vi "Display and Log Custom Device Error.vi"(7 "Error Log Settings":T1, 8 "error out":errorcluster, 9 "Note (empty)":string, 10 "Your code's public name":string, 11 "Custom Device? (T)":bool=TRUE) -> ()   [LabVIEW 2026, in "VS Inline Async API (Express).lvlib" / "VS Inline Async API (Express).lvclass"]
uses:
  VS Inline Async API (Express).lvclass
  <vilib>/NI VeriStand/Custom Device Tools/Custom Device Utility Library/Custom Device Utility Library.lvlib
  VS Inline Async API (Express).lvlib
  <vilib>/Utility/SystemLogging/NI_SystemLogging.lvlib
  <vilib>/Utility/error.llb/Trim Whitespace (string).vi
  Types/Error Handling Settings.ctl
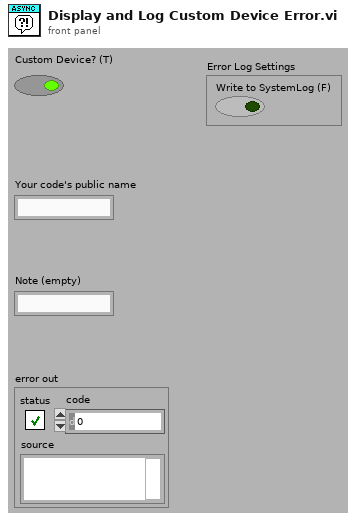
[diagram p1: front panel]
types:
  T1 = typedef "VS Inline Async API (Express).lvlib/VS Inline Async API (Express).lvclass/Error Handling Settings.ctl" = cluster{"Write to SystemLog (F)":bool}
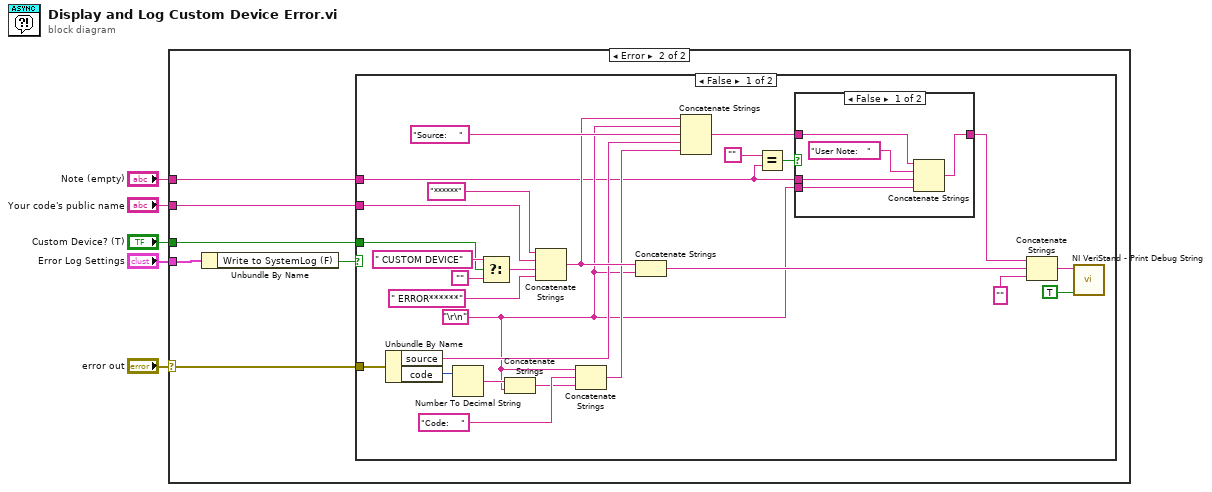
[diagram p0: block diagram]
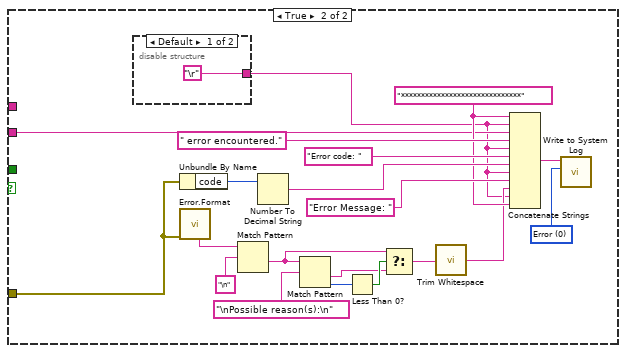
[diagram p4: hidden frame]
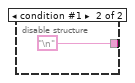
[diagram p5: hidden frame]
diagram:
  n1 = case shown="Error" "error out" {
    selector: "error out" -> [_ w11]
    tunnel: "Custom Device? (T)" -> [_ w10]
    tunnel: "Your code's public name" -> [_ w9]
    tunnel: "Note (empty)" -> [_ w8]
    tunnel: "Error Log Settings" -> [_ w7]
    frame No Error {
    }
    frame Error {
      n2 = Unbundle By Name(w7) -> ("Write to SystemLog (F)"=w6:bool)
      n3 = case shown="False" w6 {
        tunnel: w11 -> [w37 w46]
        tunnel: w10 -> [w25 _]
        tunnel: w9 -> [w16 w45]
        tunnel: w8 -> [w14 _]
        frame False {
          w15 = "\r\n"
          n4 = Unbundle By Name(w37) -> ("source"=w24:string, "code"=w18:i32)
          n5 = Number To Decimal String(number=w18) -> (decimal integer string=w34:string)  [unwired: 1 in]
          n6 = Select(t=" CUSTOM DEVICE" ("String"), s=w25, f="") -> (s? t:f=w26:string)
          n7 = Concatenate Strings(w34, w15) -> (w17:string)
          n8 = Concatenate Strings("******" ("String"), w16, w26, " ERROR******" ("String")) -> (w29:string)
          n9 = Concatenate Strings(w15, "Code:    " ("String"), w17) -> (w23:string)
          n10 = Concatenate Strings(w29, w15) -> (w20:string)
          n11 = Concatenate Strings(w29, w15, "Source:    " ("String"), w24, w23) -> (w22:string)
          n12 = Equal?(x="", y=w14) -> (x = y?=w27:bool)
          n13 = case shown="False" w27 {
            tunnel: w14 -> [w41 _]
            tunnel: w15 -> [w40 _]
            tunnel: w22 -> [w39 w43]
            tunnel: [w38 w43] -> w21
            frame False {
              n14 = Concatenate Strings(w39, "User Note:   " ("string"), w41, w40) -> (w38:string)
            }
            frame True {
            }
          }
          n15 = Concatenate Strings(w21, w20, "" ("Message")) -> (w13:string)
          n16 = call <vilib>:"NI VeriStand - Print Debug String.vi"("Add to log file? (F)"=TRUE ("Add to log file? (T)"), "Message"=w13) -> ()  [unwired: 9 in, 1 out]
        }
        frame True {
          w58 = "******************************" ("string")
          w63 = 0 items=["Error", "Warning", "Informational"] ("severity")
          n17 = disable-structure shown="Default" {
            disable-tunnel: ["\r" "\n"] -> w44
            frame condition #0 (active) {
            }
            frame condition #1 {
            }
          }
          n18 = Unbundle By Name(w46) -> ("code"=w47:i32)
          n19 = call "Error.Format.vi"("error in (no error)"=w46) -> ("message"=w48:string)  [unwired: 6 in, 4 out]
          n20 = Match Pattern(string=w48, regular expression="\n" ("string")) -> (after substring=w53:string)  [unwired: 1 in, 3 out]
          n21 = Number To Decimal String(number=w47) -> (decimal integer string=w60:string)  [unwired: 1 in]
          n22 = Match Pattern(string=w53, regular expression="\nPossible reason(s):\n" ("string")) -> (after substring=w52:string, offset past match=w55:i32)  [unwired: 1 in, 2 out]
          n23 = Less Than 0?(x=w55) -> (x < 0?=w54:bool)
          n24 = Select(t=w53, s=w54, f=w52) -> (s? t:f=w51:string)
          n25 = call-poly <vilib>:"Trim Whitespace.vi"("string"=w51) -> ("trimmed string"=w50:string)  [unwired: 1 in]
          n26 = Concatenate Strings(w58, w44, w45, " error encountered." ("String"), w44, "Error code: " ("string"), w60, w44, "Error Message: " ("string"), w50, w44, w58) -> (w49:string)
          n27 = call <vilib>:"Write to System Log.vi"("severity"=w63, "message"=w49) -> ()  [unwired: 9 in, 1 out]
        }
      }
    }
  }
